vi "Create Sysdef Tree.vi"(7 "error in (no error)":errorcluster, 10 "Device Ref":T1 format="%.0x") -> (0 "error out":errorcluster, 3 "Device Ref Out":T1 format="%.0x")   [LabVIEW 2011, in "NI 272x Resistive Simulation Custom Device Configuration.lvlib"]
uses:
  NI 272x Resistive Simulation Custom Device Configuration.lvlib
  <vilib>/NI Veristand/Custom Device API/Custom Device Item Ref.ctl
  <vilib>/NI Veristand/Custom Device API/Custom Device Channel.ctl
  <vilib>/NI Veristand/Custom Device API/Custom Device Channel Type.ctl
  Globals/Names.vi
  <vilib>/NI Veristand/Custom Device API/Set Item Property (String).vi
  NI 272x Resistive Simulation Custom Device Shared.lvlib
  <vilib>/NI Veristand/Custom Device API/Custom Device API.lvlib
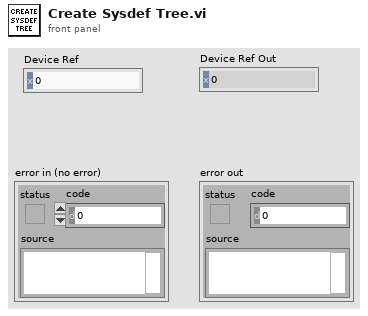
[diagram p1: front panel]
types:
  T1 = typedef "Custom Device API.lvlib/Custom Device Item Ref.ctl" = u64
  T2 = typedef "Custom Device API.lvlib/Custom Device Channel Type.ctl" = enum16{"Input", "Output"}
  T3 = typedef "Custom Device API.lvlib/Custom Device Channel.ctl" = cluster{"Type":T2, "Units":string, "Default Value":dbl, "Faultable":bool, "Scalable":bool}
  T4 = typedef "NI 272x Resistive Simulation Custom Device Shared.lvlib/Channel Mode.ctl" = enum16{"Resistance", "RTD Temperature"}
  T5 = typedef "ni272x Callendar-Van Dusen RTD Parameters.ctl" = cluster{"A":dbl, "B":dbl, "C":dbl, "R0":dbl}
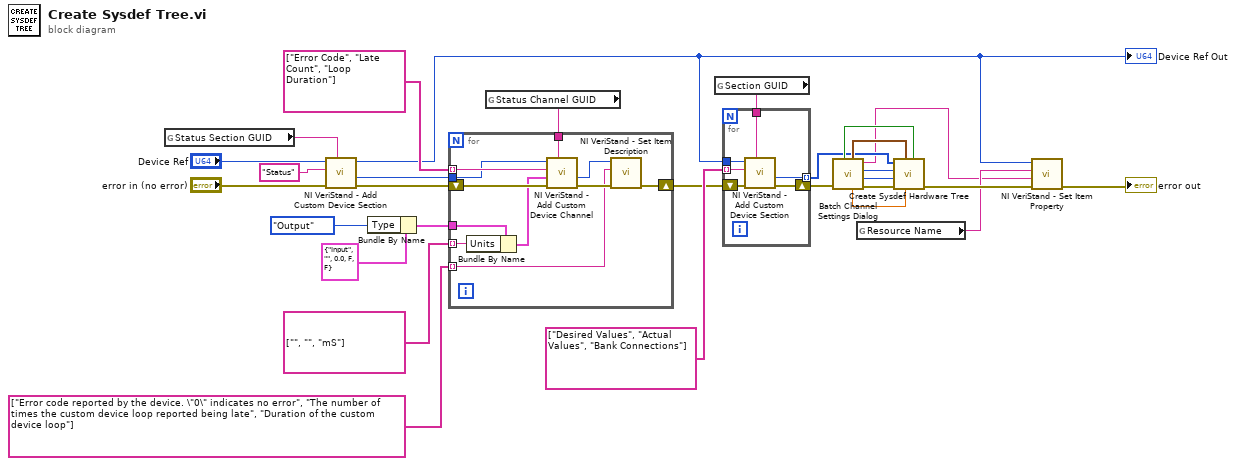
[diagram p0: block diagram]
diagram:
  n1 = global read "Names.vi" "Status Section GUID"() -> (w25:string)
  n2 = call <vilib>:"NI VeriStand - Add Custom Device Section.vi"("GUID (Default Section)"=w25, "error in (no error)"="error in (no error)", "Section Name"="Status", "Parent Ref in"="Device Ref") -> ("error out"=w20:errorcluster, "Section Ptr"=w19:T1, "Parent Ref out"=w3:T1)  [unwired: 4 in, 1 out]
  "Device Ref Out" <- w3
  n3 = Bundle By Name(cluster=T3 {"Type"=enum."Input", "Units"="", "Default Value"=0.0, "Faultable"=FALSE, "Scalable"=FALSE} ("Channel"), "Type"=Custom_Device_Channel_Type."Output") -> (w16:T3)
  n4 = global read "Names.vi" "Status Channel GUID"() -> (w11:string)
  n5 = for {
    shift-right: [w31] -> w8
    shift-left: w20 -> [w40]
    tunnel: w19 -> [w37]
    tunnel: w16 -> [w39]
    tunnel: string[] ["Error Code", "Late Count", "Loop Duration"] -> [w38] mode=indexing
    tunnel: string[] ["", "", "mS"] -> [w35] mode=indexing
    tunnel: string[] ["Error code reported by the device. \"0\" indicates no error", "The number of times the custom device loop reported being late", "Duration of the custom device loop"] -> [w32] mode=indexing
    tunnel: w11 -> [w30]
    n6 = Bundle By Name(cluster=w39, "Units"=w35) -> (w36:T3)
    n7 = call <vilib>:"NI VeriStand - Add Custom Device Channel.vi"("GUID (Default Channel)"=w30, "error in (no error)"=w40, "Channel"=w36, "Channel Name"=w38, "Parent Ref in"=w37) -> ("error out"=w34:errorcluster, "Channel Ref"=w33:T1)  [unwired: 3 in, 2 out]
    n8 = call <vilib>:"NI VeriStand - Set Item Description.vi"("error in (no error)"=w34, "Description"=w32, "Item Ref in"=w33) -> ("error out"=w31:errorcluster)  [unwired: 6 in, 2 out]
  }
  n9 = global read "Names.vi" "Section GUID"() -> (w9:string)
  n10 = for {
    tunnel: w3 -> [w45]
    tunnel: string[] ["Desired Values", "Actual Values", "Bank Connections"] -> [w44] mode=indexing
    tunnel: w9 -> [w43]
    shift-right: [w42] -> w7
    shift-left: w8 -> [w46]
    tunnel: [w41] -> w6 mode=indexing
    n11 = call <vilib>:"NI VeriStand - Add Custom Device Section.vi"("GUID (Default Section)"=w43, "error in (no error)"=w46, "Section Name"=w44, "Parent Ref in"=w45) -> ("error out"=w42:errorcluster, "Section Ptr"=w41:T1)  [unwired: 4 in, 2 out]
  }
  n12 = call "Batch Channel Settings Dialog.vi"("error in (no error)"=w7) -> ("error out"=w26:errorcluster, "Mode selected"=w27:T4, "channels selected"=w28:i32, "Selected name"=w1:string, "Default Value"=w5:dbl, "Temp params"=w29:T5, "Create bank channels"=w12:bool)  [unwired: 4 in]
  n13 = global read "Names.vi" "Resource Name"() -> (w2:string)
  n14 = call "Create Sysdef Hardware Tree.vi"("Create bank channels"=w12, "Default Value"=w5, "temp param"=w29, "Error In"=w26, "Mode"=w27, "number of channels"=w28, "Section Refs"=w6) -> ("Error Out"=w23:errorcluster)  [unwired: 4 in]
  n15 = call-poly <vilib>:"NI VeriStand - Set Item Property.vi"("error in (no error)"=w23, "Value"=w1, "Property Name"=w2, "Item Ref in"=w3) -> ("error out"=→"error out":errorcluster)  [unwired: 5 in, 2 out]
